vi "onSerializeHeaderString.vi"(8 "error in (no error)":errorcluster, 10 "headers":cluster{"header":string, "value":string}[](array[cluster]), 11 "httpHeaders":refnum<class "httpHeaders.lvclass">) -> (0 "error out":errorcluster, 2 "http-header":string)   [LabVIEW 2020, in "httpClient.lvlib" / "httpHeaders.lvclass"]
uses:
  httpHeaders.lvclass
  httpHeaders.lvclass/httpHeaders.ctl
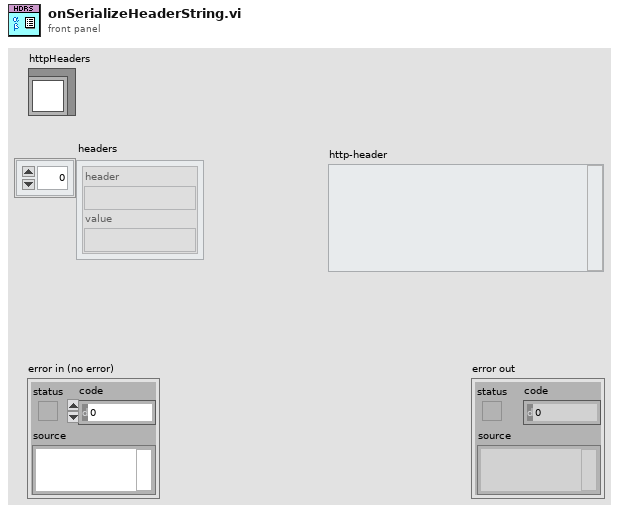
[diagram p1: front panel]
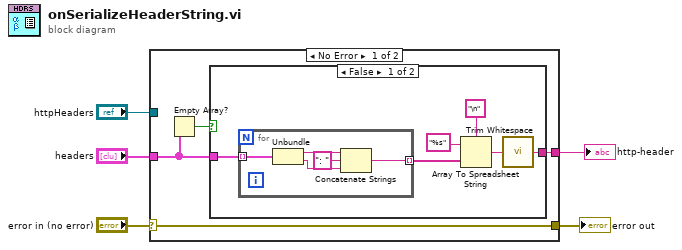
[diagram p0: block diagram]
diagram:
  n1 = case shown="No Error" "error in (no error)" {
    selector: "error in (no error)" -> [w9 w21]
    tunnel: [w9 w21] -> w4
    tunnel: "httpHeaders" -> [_ _]
    tunnel: "headers" -> [w7 _]
    tunnel: [w8 _] -> w1
    frame No Error {
      n2 = Empty Array?(array=w7) -> (empty?=w6:bool)
      n3 = case shown="False" w6 {
        tunnel: [w11 _] -> w8
        tunnel: w7 -> [w10 _]
        frame False {
          n4 = for {
            tunnel: w10 -> [w20] mode=indexing
            tunnel: [w17] -> w15 mode=indexing
            n5 = Unbundle(w20) -> ("header"=w19:string, "value"=w16:string)
            n6 = Concatenate Strings(w19, ": " ("string"), w16) -> (w17:string)
          }
          n7 = Array To Spreadsheet String(delimiter (Tab)="\n", array=w15, 3:"%s" ("format string")) -> (spreadsheet string=w12:string)
          n8 = call <vilib>:"Trim Whitespace.vi"("string"=w12) -> ("trimmed string"=w11:string)  [unwired: 1 in]
        }
        frame True {
        }
      }
    }
    frame Error {
    }
  }
  "error out" <- w4
  "http-header" <- w1
